vi "Initialize HW.vi"(8 "error in (no error)":errorcluster, 11 "General Hardware in":refnum<class "General Hardware.lvclass">) -> (0 "error out":errorcluster, 3 "General Hardware out":refnum<class "General Hardware.lvclass">)   [LabVIEW 2020, in "General Hardware.lvclass"]
uses:
  General Hardware.lvclass
  General Hardware.lvclass/General Hardware.ctl
panel:
  in  "frequency (Hz)":dbl
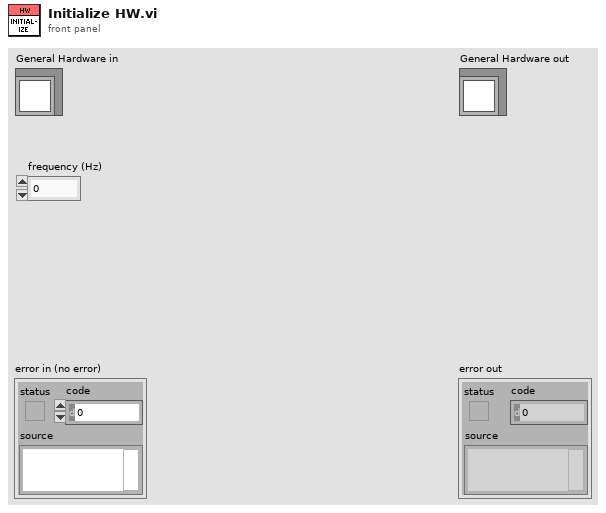
[diagram p1: front panel]
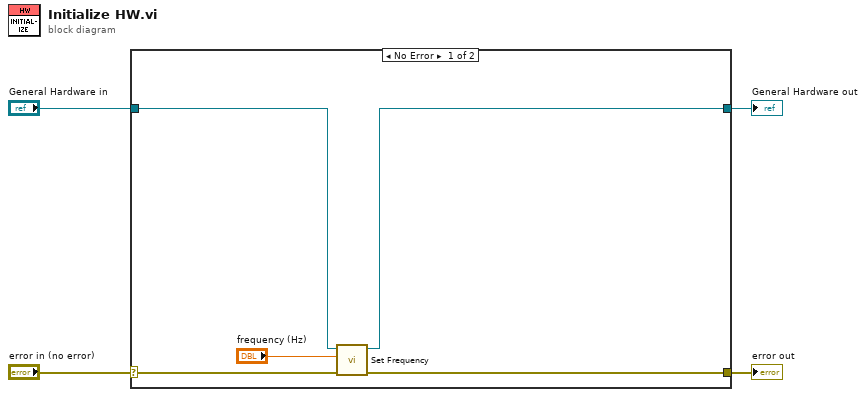
[diagram p0: block diagram]
diagram:
  n1 = case shown="No Error" "error in (no error)" {
    selector: "error in (no error)" -> [w8 w11]
    tunnel: [w7 w11] -> w3
    tunnel: [w5 w10] -> w1
    tunnel: "General Hardware in" -> [w6 w10]
    frame No Error {
      n2 = call "Set Frequency.vi"("error in (no error)"=w8, "frequency (Hz)"="frequency (Hz)", "General Hardware in"=w6) -> ("error out"=w7:errorcluster, "General Hardware out"=w5:refnum<class "General Hardware.lvclass">)  [unwired: 7 in]
    }
    frame Error {
    }
  }
  "error out" <- w3
  "General Hardware out" <- w1
